vi "Utility Default Instrument Setup.vi"(0 "VISA resource name":refnum<visa-resource-name>, 11 "error in (no error)":errorcluster) -> (4 "VISA resource name out":refnum<visa-resource-name>, 15 "error out":errorcluster)   [LabVIEW 2013, in "Yokogawa WT200 Series.lvlib"]
doc: "This Utility VI sends a default command string to the instrument whenever a new VISA session is opened, or the instrument is reset. This VI is intended to be used as a subVI for the YKWT200 Initialize and YKWT200 Reset VI's. Altering this VI could cause these two VI's to operate incorrectly."
uses:
  <instrlib>/Yokogawa WT200 Series/Yokogawa WT200 Series.lvlib
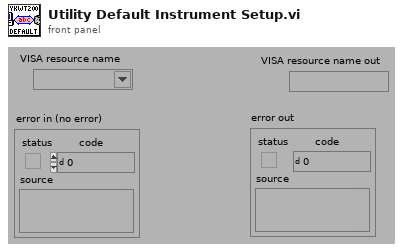
[diagram p1: front panel]
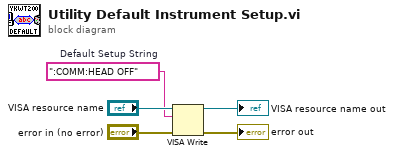
[diagram p0: block diagram]
diagram:
  w1 = ":COMM:HEAD OFF"  # Default Setup String
  n1 = VISA Write(VISA resource name="VISA resource name", write buffer=w1, error in (no error)="error in (no error)") -> (VISA resource name out=→"VISA resource name out":refnum<visa-resource-name>, error out=→"error out":errorcluster)  [unwired: 1 out]
